vi "AutoInit.vi"(7 "AutoMode":T1, 8 "error in (no error)":errorcluster, 9 "BallSettleWait":u32, 11 "StartInLowGear?":bool) -> (0 "error out":errorcluster)   [LabVIEW 2013]
uses:
  AutoMode.ctl
  SingleSolenoidAction.ctl
  DoubleSolenoidAction.ctl
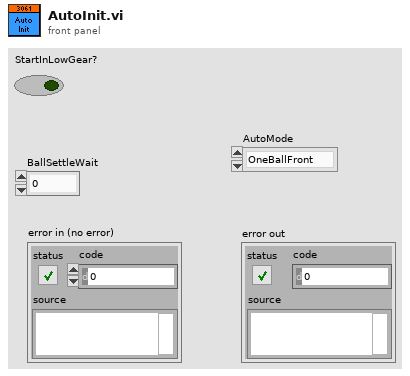
[diagram p1: front panel]
types:
  T1 = typedef "AutoMode.ctl" = enum16{"OneBallFront", "OneBallCollector", "TwoBallNormal", "TwoBallHot"}
  T2 = typedef "DoubleSolenoidAction.ctl" = enum16{"Init", "Middle", "In", "Out"}
  T3 = typedef "SingleSolenoidAction.ctl" = enum16{"Init", "SetState", "Disable"}
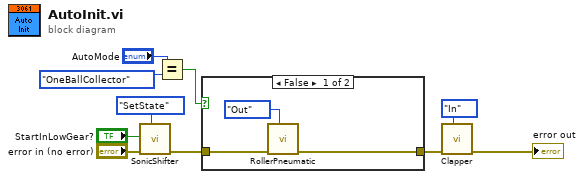
[diagram p0: block diagram]
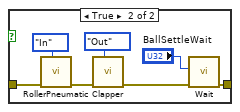
[diagram p2: hidden frame]
diagram:
  n1 = call "SonicShifter.vi"("Action"=SingleSolenoidAction."SetState", "error in (no error)"="error in (no error)", "Actuate?"="StartInLowGear?") -> ("error out"=w7:errorcluster)  [unwired: 8 in]
  n2 = Equal?(x="AutoMode", y=AutoMode."OneBallCollector") -> (x = y?=w5:bool)
  n3 = case shown="False" w5 {
    tunnel: [w12 w15] -> w8
    tunnel: w7 -> [w11 w16]
    frame False {
      n4 = call "RollerPneumatic.vi"("State"=DoubleSolenoidAction."Out", "Error in"=w11) -> ("Error out"=w12:errorcluster)  [unwired: 9 in]
    }
    frame True {
      n5 = call "RollerPneumatic.vi"("State"=DoubleSolenoidAction."In", "Error in"=w16) -> ("Error out"=w17:errorcluster)  [unwired: 9 in]
      n6 = call "Clapper.vi"("State"=DoubleSolenoidAction."Out", "Error in"=w17) -> ("Error out"=w19:errorcluster)  [unwired: 9 in]
      n7 = call "Wait.vi"("error in"=w19, "milliseconds to wait"="BallSettleWait") -> ("error out"=w15:errorcluster)  [unwired: 9 in]
    }
  }
  n8 = call "Clapper.vi"("State"=DoubleSolenoidAction."In", "Error in"=w8) -> ("Error out"=→"error out":errorcluster)  [unwired: 9 in]
